vi "send_to_watchdog.vi"(8 "error in":errorcluster, 9 "Process_name":string(combo), 10 "Feedback_from_process_enum in":T1, 11 "Process_communication in":variant) -> (0 "error out":errorcluster, 3 "Process_communication out":variant)   [LabVIEW 2011, in "Fiberscope_library.lvlib"]
uses:
  Fiberscope_library.lvlib
  typedefs/feedback_from_process_enum.ctl
  typedefs/feedback_to_watchdog.ctl
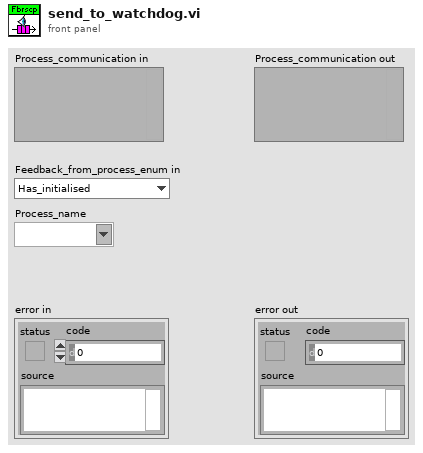
[diagram p1: front panel]
types:
  T1 = typedef "Fiberscope_library.lvlib/feedback_from_process_enum.ctl" = enum16{"Has_initialised", "Changed_parameters", "Has_started", "Has_stopped", "Has_quitted", "Is_running", "Has_finished", "Custom"}
  T2 = typedef "Fiberscope_library.lvlib/feedback_to_watchdog.ctl" = cluster{"Feedback_from_process_enum":T1, "Process_name":string}
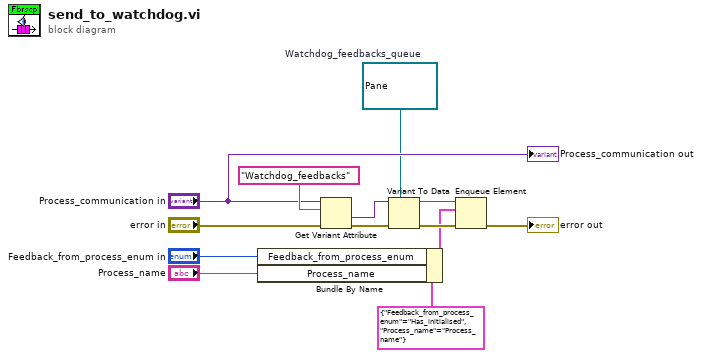
[diagram p0: block diagram]
diagram:
  w5 = refnum<queue> refnum  # Watchdog_feedbacks_queue
  n1 = Bundle By Name(cluster=T2 {"Feedback_from_process_enum"=enum."Has_initialised", "Process_name"="Process_name"} ("Feedback_to_watchdog"), "Feedback_from_process_enum"="Feedback_from_process_enum in", "Process_name"="Process_name") -> (w1:T2)
  n2 = Get Variant Attribute(Variant="Process_communication in", name="Watchdog_feedbacks", error in="error in") -> (value=w8:variant, error out=w12:errorcluster)  [unwired: 1 in, 2 out]
  n3 = Variant To Data(error in=w12, type=w5, Variant=w8) -> (data=w7:refnum<queue>, error out=w13:errorcluster)
  n4 = Enqueue Element(queue=w7, element=w1, error in (no error)=w13) -> (error out=→"error out":errorcluster)  [unwired: 1 in, 2 out]
  "Process_communication out" <- "Process_communication in"
